vi "Dock Window.vi"(0 "Py Doc in":refnum<class "Py Doc.lvclass">, 5 "Dock?":bool, 7 "Parent Hwnd":i32, 11 "error in (no error)":errorcluster) -> (4 "Py Doc out":refnum<class "Py Doc.lvclass">, 15 "error out":errorcluster)   [LabVIEW 2016, in "Py Doc.lvclass"]
uses:
  Py Doc.lvclass
  D:/MDI Project/source code/Document/Document.lvclass
  Document.lvclass/Document.ctl
  Py Doc.lvclass/Py Doc.ctl
  user32.dll
  Document.lvclass
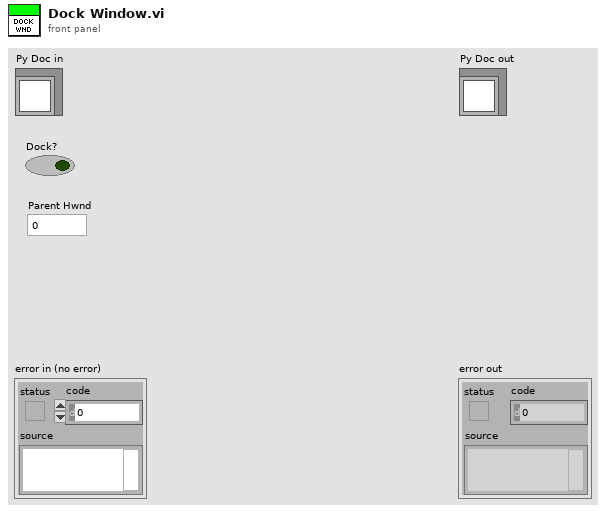
[diagram p1: front panel]
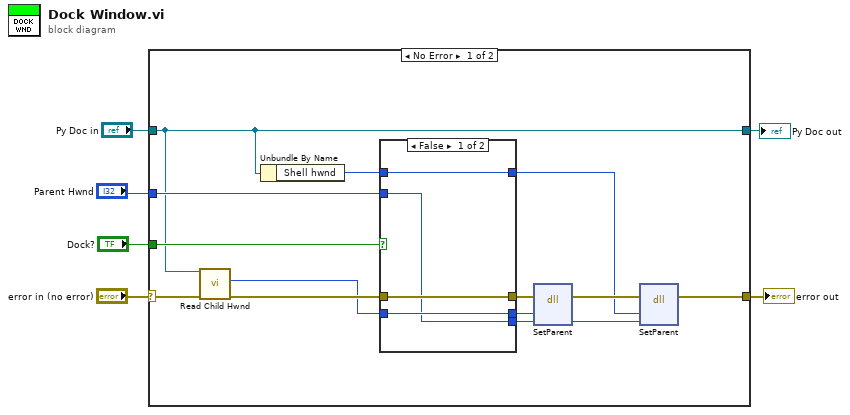
[diagram p0: block diagram]
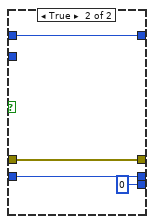
[diagram p2: hidden frame]
diagram:
  n1 = case shown="No Error" "error in (no error)" {
    selector: "error in (no error)" -> [w15 w30]
    tunnel: [w9 w30] -> w5
    tunnel: "Py Doc in" -> [w12 w29]
    tunnel: [w12 w29] -> w3
    tunnel: "Dock?" -> [w14 _]
    tunnel: "Parent Hwnd" -> [w13 _]
    frame No Error {
      n2 = call "Read Child Hwnd.vi"("error in (no error)"=w15, "Document in"=w12) -> ("error out"=w17:errorcluster, "Child Hwnd"=w16:u32)  [unwired: 7 in, 1 out]
      n3 = Unbundle By Name(w12) -> ("Shell hwnd"=w11:u32)
      n4 = case shown="False" w14 {
        tunnel: w17 -> [w24 w28]
        tunnel: [w24 w28] -> w20
        tunnel: [w23 w27] -> w19
        tunnel: [w22 0 ("hWnd")] -> w18
        tunnel: w16 -> [w23 w27]
        tunnel: w13 -> [w22 _]
        tunnel: w11 -> [w21 w25]
        tunnel: [w21 w25] -> w7
        frame False {
        }
        frame True {
        }
      }
      n5 = dll-call lib="user32.dll" fn="SetParent"(error in=w20, "Child"=w19, "NewParent"=w18) -> (error out=w10:errorcluster, "NewParent"=w8:i32)  [unwired: 4 in, 1 out]
      n6 = dll-call lib="user32.dll" fn="SetParent"(error in=w10, "Child"=w7, "NewParent"=w8) -> (error out=w9:errorcluster)  [unwired: 5 in, 1 out]
    }
    frame Error {
    }
  }
  "error out" <- w5
  "Py Doc out" <- w3
